vi "Set Node Badge.vi"(0 "FSM in":refnum<class "FSM.Graph.lvclass">, 5 "nodeIndex":i32, 7 "Badge":T1, 9 "visible":bool, 11 "error in (no error)":errorcluster) -> (4 "FSM out":refnum<class "FSM.Graph.lvclass">, 15 "error out":errorcluster)   [LabVIEW 2015, in "FSM.Graph.lvclass"]
uses:
  FSM.Graph.lvclass
  FSM.Node/Badge.ctl
  FSM.Graph.lvclass/FSM.Graph.ctl
  FSM.Node/FSM.Node.lvclass
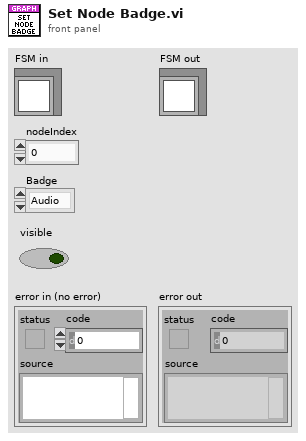
[diagram p1: front panel]
types:
  T1 = typedef "FSM.Node.lvclass/Badge.ctl" = enum16{"Audio", "Visual"}
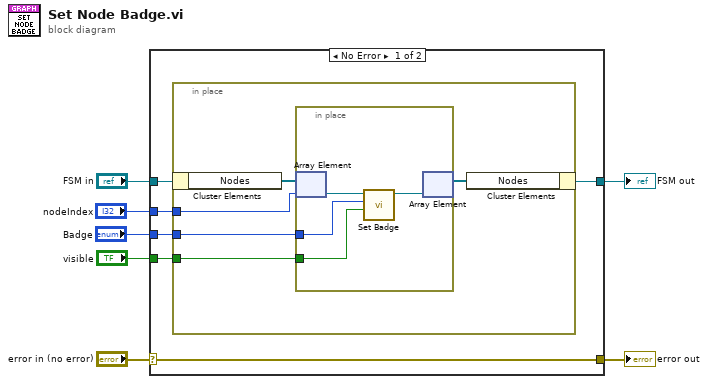
[diagram p0: block diagram]
diagram:
  n1 = case shown="No Error" "error in (no error)" {
    selector: "error in (no error)" -> [w13 w24]
    tunnel: [w13 w24] -> w6
    tunnel: [w10 w23] -> w4
    tunnel: "FSM in" -> [w12 w23]
    tunnel: "nodeIndex" -> [w11 _]
    tunnel: "visible" -> [w9 _]
    tunnel: "Badge" -> [w8 _]
    frame No Error {
      n2 = in-place {
        in-place-border: w11 -> [w17]
        in-place-border: w9 -> [w15]
        in-place-border: w8 -> [w14]
        n3 = in-place-cluster #1(w12) -> ("Nodes"=w18:refnum<class "FSM.Node.lvclass">[])
        n4 = in-place {
          in-place-border: w15 -> [w20]
          in-place-border: w14 -> [w21]
          n5 = in-place-array #2(w18, w17) -> (w22:refnum<class "FSM.Node.lvclass">)
          n6 = call "Set Badge.vi"("visible"=w20, "Badge"=w21, "FSM in"=w22) -> ("FSM out"=w19:refnum<class "FSM.Node.lvclass">)  [unwired: 7 in, 1 out]
          n7 = in-place-array #2(w19) -> (w16:refnum<class "FSM.Node.lvclass">[])  [unwired: 1 out]
        }
        n8 = in-place-cluster #1("Nodes"=w16) -> (w10:refnum<class "FSM.Graph.lvclass">)
      }
    }
    frame Error {
    }
  }
  "error out" <- w6
  "FSM out" <- w4
